vi "Open Comm Port V.vi"(8 "error in (no error)":errorcluster, 10 "baudRate":i32, 11 "comPort":i16) -> (0 "error out":errorcluster, 3 "function return":i16)   [LabVIEW 2012, in "VantagePro.lvlib"]
doc: "DllAccess short int _stdcall OpenCommPort_V (short int comPort, int baudRate);"
uses:
  VantagePro.lvlib
  VantagePro.dll
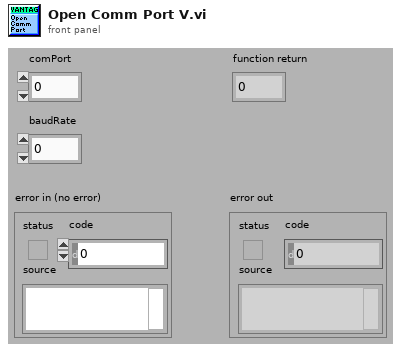
[diagram p1: front panel]
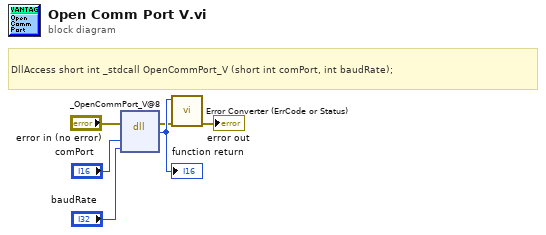
[diagram p0: block diagram]
diagram:
  # "DllAccess short int _stdcall OpenCommPort_V (short int comPort, int baudRate);"
  n1 = dll-call lib="C:/Users/Dimitris/Desktop/BRITE/libs/VantagePro/VantagePro.*" fn="_OpenCommPort_V@8"(error in="error in (no error)", "comPort"="comPort", "baudRate"="baudRate") -> (error out=w2:errorcluster, w6:i16)  [unwired: 4 in, 1 out]
  "function return" <- w6
  n2 = call "Error Converter (ErrCode or Status).vi"("error in (no error)"=w2, "error code"=w6) -> ("error out"=→"error out":errorcluster)  [unwired: 9 in]
